vi "AutoFit.vi"(8 "error":errorcluster caption="错误输入（无错误）", 9 "水平？":bool, 10 "垂直？":bool, 11 "Excel._Worksheet":refnum<k7>) -> (0 "error out":errorcluster caption="错误输出", 3 "Excel._Worksheet":refnum<k7>)   [LabVIEW 2017]
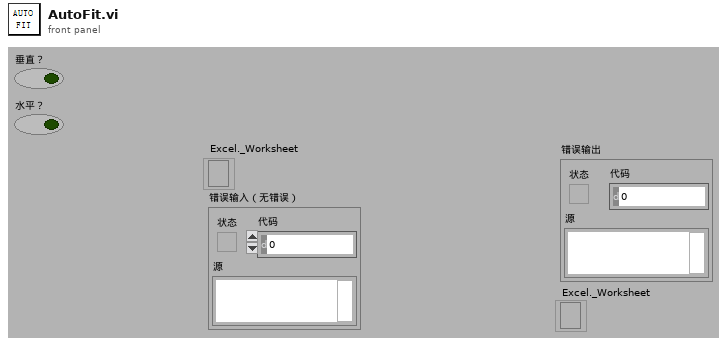
[diagram p1: front panel]
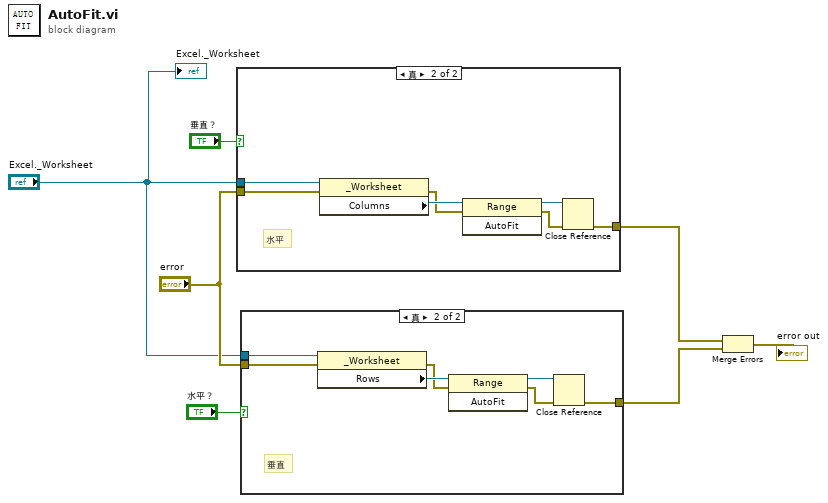
[diagram p0: block diagram]
diagram:
  n1 = case shown="真" "垂直？" {
    tunnel: "Excel._Worksheet" -> [_ w15]
    tunnel: [w8 w10] -> w4
    tunnel: "error" -> [w8 w9]
    frame False {
    }
    frame True {
      # "水平"
      n2 = property class="_Worksheet"(reference=w15, error in=w9) -> (error out=w11:errorcluster, "Columns"=w14:refnum<k7>)  [unwired: 1 out]
      n3 = invoke class="Range" method="AutoFit"(reference=w14, error in=w11) -> (reference out=w13:refnum<k7>, error out=w12:errorcluster)  [unwired: 1 in, 1 out]
      n4 = Close Reference(reference=w13, error in (no error)=w12) -> (error out=w10:errorcluster)
    }
  }
  n5 = case shown="真" "水平？" {
    tunnel: "Excel._Worksheet" -> [_ w23]
    tunnel: [w16 w18] -> w3
    tunnel: "error" -> [w16 w17]
    frame False {
    }
    frame True {
      # "垂直"
      n6 = property class="_Worksheet"(reference=w23, error in=w17) -> (error out=w19:errorcluster, "Rows"=w22:refnum<k7>)  [unwired: 1 out]
      n7 = invoke class="Range" method="AutoFit"(reference=w22, error in=w19) -> (reference out=w21:refnum<k7>, error out=w20:errorcluster)  [unwired: 1 in, 1 out]
      n8 = Close Reference(reference=w21, error in (no error)=w20) -> (error out=w18:errorcluster)
    }
  }
  n9 = Merge Errors(w4, w3) -> (→"error out":errorcluster)
  "Excel._Worksheet" <- "Excel._Worksheet"
